vi "WVDIAL_1_MCSC_v1.vi"() -> ()   [LabVIEW 2012]
uses:
  <vilib>/Analysis/baseanly.llb/Mean (DBL).vi
  H2O_DIAL/LabVIEW-2012/Scalar_Data.vi
  AmcsUsb.dll
  <vilib>/Analysis/NI_AALBase.lvlib
panel:
  in  "Near Ch Offline mult":dbl=2.6
  in  "Data Reads":i32=770
  out "Loop Count":i32=770
  in  "TC Start":i32=100 min=1 max=1894
  in  "TC Length":i32=190 min=100 max=1894
  out "Total Counts":cluster{dbl, dbl, dbl, dbl}(graph)={168433.0, 167767.0, 1145442.0, 1147692.0}
  out "return type":i32
  out "Raw Uncorrected Return":dbl[][](graph)=[[20897.0, 17907.0, 61299.0, 1003.0, 932.0, 983.0, 951.0, 944.0, 1016.0, 1068.0, 1049.0, 1010.0, 1053.0, 979.0, 1043.0, 1051.0, 1088.0, 1105.0, 1050.0, 1051.0, 1029.0, 1012.0, 1012.0, 1067.0, 1114.0, 1055.0, 993.0, 1021.0, 944.0, 1017.0, 1050.0, 1058.0, 988.0, 1006.0, 985.0, 995.0, 1349.0, 2765.0, 4753.0, 5334.0, 4567.0, 3771.0, 2737.0, 1942.0, 1415.0, 1577.0, 1781.0, 1958.0, 1989.0, 1616.0, 5808.0, 11417.0, 8373.0, 1568.0, 979.0, 935.0, 900.0, 910.0, 923.0, 946.0, 962.0, 941.0, 927.0, 963.0, 943.0, 965.0, 941.0, 987.0, 993.0, 1007.0, 1151.0, 1083.0, 982.0, 1005.0, 997.0, 1039.0, 986.0, 980.0, 893.0, 968.0, 991.0, 1035.0, 1066.0, 1129.0, 1065.0, 1035.0, 926.0, 1000.0, 1000.0, 976.0, 914.0, 944.0, 888.0, 970.0, 917.0, 937.0, 943.0, 953.0, 866.0, 863.0, 952.0, 900.0, 961.0, 913.0, 941.0, 971.0, 946.0, 917.0, 939.0, 926.0, 944.0, 975.0, 937.0, 915.0, 916.0, 892.0, 900.0, 955.0, 938.0, 902.0, 912.0, 961.0, 927.0, 893.0, 938.0, 950.0, 882.0, 872.0, 953.0, 967.0, 902.0, 955.0, 932.0, 912.0, 969.0, 955.0, 951.0, 945.0, 994.0, 952.0, 949.0, 977.0, 917.0, 930.0, 888.0, 951.0, 935.0, 896.0, 923.0, 863.0, 979.0, 900.0, 1008.0, 893.0, 929.0, 917.0, 920.0, 943.0, 949.0, 881.0, 981.0, 916.0, 937.0, 911.0, 932.0, 945.0, 976.0, 882.0, 911.0, 994.0, 969.0, 919.0, 971.0, 898.0, 923.0, 930.0, 947.0, 904.0, 982.0, 933.0, 914.0, 970.0, 977.0, 881.0, 959.0, 947.0, 899.0, 949.0, 942.0, 951.0, 919.0, 910.0, 944.0, 931.0, 967.0, 901.0, 922.0, 921.0, 984.0, 977.0, 932.0, 906.0, 972.0, 872.0, 887.0, 920.0, 983.0, 1002.0, 945.0, 948.0, 897.0, 925.0, 965.0, 955.0, 909.0, 933.0, 953.0, 924.0, 972.0, 964.0, 961.0, 1002.0, 966.0, 904.0, 899.0, 951.0, 944.0, 938.0, 993.0, 893.0, 1016.0, 900.0, 879.0, 876.0, 944.0, 889.0, 935.0, 924.0, 961.0, 931.0, 933.0, 926.0, 862.0, 958.0, 885.0, 978.0, 968.0, 1002.0, 875.0, 912.0, 971.0, 922.0, 979.0, 959.0, 917.0, 971.0, 940.0, 891.0, 976.0, 932.0, 893.0, 934.0, 922.0, 989.0, 959.0, 932.0, 954.0, 947.0, 895.0, 950.0, 946.0, 943.0, 902.0, 911.0, 919.0, 1012.0, 904.0, 918.0, 965.0, 975.0], [922.0, 18275.0, 62214.0, 993.0, 957.0, 995.0, 1005.0, 1002.0, 1103.0, 1102.0, 1143.0, 1148.0, 1161.0, 1218.0, 1193.0, 1189.0, 1300.0, 1250.0, 1305.0, 1319.0, 1301.0, 1306.0, 1275.0, 1325.0, 1316.0, 1250.0, 1254.0, 1267.0, 1215.0, 1264.0, 1260.0, 1198.0, 1209.0, 1132.0, 1074.0, 1284.0, 2617.0, 7789.0, 14632.0, 16266.0, 14395.0, 11311.0, 8121.0, 5107.0, 3254.0, 3555.0, 4576.0, 5500.0, 5467.0, 4251.0, 20644.0, 36289.0, 27186.0, 3510.0, 957.0, 934.0, 965.0, 975.0, 950.0, 925.0, 944.0, 975.0, 978.0, 930.0, 906.0, 972.0, 923.0, 967.0, 1148.0, 1539.0, 1778.0, 1640.0, 1402.0, 1251.0, 1253.0, 1337.0, 1313.0, 1092.0, 1182.0, 1150.0, 1259.0, 1458.0, 1826.0, 1997.0, 1783.0, 1387.0, 1119.0, 1085.0, 1015.0, 951.0, 912.0, 947.0, 945.0, 935.0, 941.0, 910.0, 901.0, 897.0, 904.0, 895.0, 947.0, 962.0, 900.0, 1009.0, 902.0, 929.0, 908.0, 957.0, 926.0, 962.0, 886.0, 920.0, 978.0, 851.0, 975.0, 885.0, 895.0, 891.0, 932.0, 945.0, 937.0, 949.0, 907.0, 961.0, 933.0, 943.0, 921.0, 891.0, 970.0, 897.0, 927.0, 882.0, 911.0, 890.0, 918.0, 937.0, 944.0, 946.0, 946.0, 981.0, 967.0, 947.0, 969.0, 931.0, 967.0, 902.0, 946.0, 943.0, 987.0, 946.0, 945.0, 893.0, 956.0, 976.0, 955.0, 915.0, 885.0, 892.0, 921.0, 912.0, 952.0, 919.0, 940.0, 939.0, 959.0, 949.0, 943.0, 918.0, 927.0, 948.0, 965.0, 975.0, 926.0, 966.0, 963.0, 873.0, 939.0, 911.0, 911.0, 924.0, 904.0, 903.0, 944.0, 955.0, 928.0, 919.0, 934.0, 957.0, 907.0, 954.0, 901.0, 958.0, 897.0, 920.0, 899.0, 865.0, 891.0, 916.0, 938.0, 913.0, 918.0, 939.0, 921.0, 918.0, 917.0, 958.0, 931.0, 901.0, 962.0, 952.0, 909.0, 973.0, 910.0, 938.0, 927.0, 875.0, 909.0, 929.0, 944.0, 889.0, 910.0, 954.0, 882.0, 1028.0, 930.0, 964.0, 972.0, 955.0, 884.0, 897.0, 982.0, 990.0, 950.0, 997.0, 944.0, 923.0, 959.0, 932.0, 940.0, 881.0, 939.0, 911.0, 882.0, 939.0, 915.0, 910.0, 954.0, 900.0, 901.0, 917.0, 893.0, 923.0, 856.0, 962.0, 948.0, 949.0, 936.0, 912.0, 993.0, 946.0, 925.0, 947.0, 907.0, 942.0, 919.0, 960.0, 938.0, 910.0, 970.0, 926.0, 918.0, 977.0, 913.0, 956.0, 1017.0, 914.0, 896.0, 967.0, 958.0, 971.0], [901.0, 17238.0, 63738.0, 6571.0, 6627.0, 6967.0, 7037.0, 6952.0, 7011.0, 7085.0, 6916.0, 6955.0, 6689.0, 6750.0, 6599.0, 6621.0, 6454.0, 6505.0, 6415.0, 6424.0, 6268.0, 6518.0, 6408.0, 6477.0, 6500.0, 6370.0, 6334.0, 6434.0, 6392.0, 6309.0, 6236.0, 6430.0, 6473.0, 6304.0, 6382.0, 6382.0, 6442.0, 6892.0, 7617.0, 7974.0, 7667.0, 7436.0, 6895.0, 6739.0, 6455.0, 6647.0, 6742.0, 6717.0, 6663.0, 6624.0, 8201.0, 10372.0, 9200.0, 6714.0, 6266.0, 6292.0, 6417.0, 6314.0, 6468.0, 6234.0, 6317.0, 6307.0, 6331.0, 6281.0, 6488.0, 6596.0, 6326.0, 6351.0, 6400.0, 6372.0, 6588.0, 6340.0, 6501.0, 6412.0, 6397.0, 6327.0, 6430.0, 6407.0, 6300.0, 6410.0, 6250.0, 6385.0, 6411.0, 6512.0, 6402.0, 6362.0, 6367.0, 6405.0, 6382.0, 6281.0, 6268.0, 6347.0, 6348.0, 6282.0, 6292.0, 6409.0, 6275.0, 6302.0, 6415.0, 6451.0, 6367.0, 6295.0, 6437.0, 6473.0, 6337.0, 6355.0, 6512.0, 6531.0, 6283.0, 6269.0, 6368.0, 6344.0, 6443.0, 6369.0, 6353.0, 6385.0, 6425.0, 6409.0, 6377.0, 6322.0, 6353.0, 6410.0, 6508.0, 6432.0, 6298.0, 6322.0, 6420.0, 6301.0, 6325.0, 6279.0, 6361.0, 6224.0, 6237.0, 6273.0, 6424.0, 6416.0, 6355.0, 6469.0, 6373.0, 6349.0, 6311.0, 6368.0, 6282.0, 6355.0, 6237.0, 6397.0, 6338.0, 6287.0, 6364.0, 6378.0, 6295.0, 6332.0, 6342.0, 6137.0, 6260.0, 6253.0, 6331.0, 6303.0, 6393.0, 6325.0, 6329.0, 6517.0, 6423.0, 6344.0, 6284.0, 6385.0, 6362.0, 6389.0, 6357.0, 6402.0, 6446.0, 6402.0, 6361.0, 6328.0, 6470.0, 6458.0, 6454.0, 6466.0, 6453.0, 6293.0, 6483.0, 6398.0, 6271.0, 6379.0, 6351.0, 6323.0, 6291.0, 6350.0, 6366.0, 6509.0, 6445.0, 6334.0, 6295.0, 6337.0, 6310.0, 6311.0, 6417.0, 6356.0, 6309.0, 6411.0, 6380.0, 6260.0, 6532.0, 6352.0, 6394.0, 6461.0, 6402.0, 6391.0, 6400.0, 6353.0, 6339.0, 6360.0, 6365.0, 6437.0, 6335.0, 6297.0, 6511.0, 6365.0, 6283.0, 6384.0, 6464.0, 6297.0, 6291.0, 6346.0, 6384.0, 6355.0, 6530.0, 6417.0, 6334.0, 6364.0, 6340.0, 6344.0, 6367.0, 6388.0, 6356.0, 6285.0, 6258.0, 6281.0, 6322.0, 6328.0, 6406.0, 6450.0, 6343.0, 6354.0, 6275.0, 6425.0, 6245.0, 6236.0, 6392.0, 6339.0, 6318.0, 6406.0, 6458.0, 6358.0, 6344.0, 6388.0, 6304.0, 6356.0, 6277.0, 6408.0, 6439.0, 6308.0, 6440.0, 6412.0, 6283.0, 6365.0, 6320.0, 6403.0, 6318.0, 6412.0, 6326.0, 6403.0, 6439.0, 6369.0, 6437.0, 6351.0, 6319.0, 6382.0, 6454.0, 6288.0], [6387.0, 17467.0, 65418.0, 6569.0, 6883.0, 7052.0, 7265.0, 7267.0, 7422.0, 7428.0, 7449.0, 7216.0, 7212.0, 7028.0, 7067.0, 6796.0, 6717.0, 6721.0, 6668.0, 6585.0, 6511.0, 6639.0, 6441.0, 6629.0, 6525.0, 6450.0, 6456.0, 6381.0, 6453.0, 6451.0, 6380.0, 6479.0, 6424.0, 6473.0, 6587.0, 6463.0, 6806.0, 8963.0, 11686.0, 12297.0, 11494.0, 10217.0, 8973.0, 7870.0, 7087.0, 7226.0, 7776.0, 8067.0, 7957.0, 7562.0, 14612.0, 22974.0, 18051.0, 7202.0, 6396.0, 6350.0, 6276.0, 6334.0, 6252.0, 6328.0, 6420.0, 6377.0, 6390.0, 6417.0, 6109.0, 6349.0, 6440.0, 6362.0, 6392.0, 6574.0, 6721.0, 6603.0, 6431.0, 6561.0, 6489.0, 6579.0, 6553.0, 6384.0, 6426.0, 6566.0, 6460.0, 6546.0, 6644.0, 6799.0, 6611.0, 6466.0, 6404.0, 6440.0, 6429.0, 6422.0, 6470.0, 6469.0, 6344.0, 6403.0, 6356.0, 6332.0, 6325.0, 6357.0, 6387.0, 6302.0, 6368.0, 6319.0, 6370.0, 6280.0, 6314.0, 6284.0, 6539.0, 6299.0, 6473.0, 6404.0, 6434.0, 6321.0, 6398.0, 6364.0, 6362.0, 6331.0, 6194.0, 6478.0, 6333.0, 6361.0, 6353.0, 6462.0, 6312.0, 6339.0, 6442.0, 6356.0, 6323.0, 6326.0, 6156.0, 6417.0, 6400.0, 6307.0, 6432.0, 6475.0, 6443.0, 6344.0, 6491.0, 6349.0, 6424.0, 6413.0, 6400.0, 6355.0, 6257.0, 6390.0, 6370.0, 6310.0, 6401.0, 6381.0, 6368.0, 6334.0, 6345.0, 6308.0, 6398.0, 6468.0, 6360.0, 6383.0, 6282.0, 6362.0, 6426.0, 6223.0, 6353.0, 6331.0, 6316.0, 6430.0, 6376.0, 6238.0, 6391.0, 6473.0, 6431.0, 6212.0, 6449.0, 6320.0, 6221.0, 6424.0, 6517.0, 6326.0, 6446.0, 6387.0, 6435.0, 6374.0, 6360.0, 6343.0, 6251.0, 6365.0, 6487.0, 6334.0, 6413.0, 6253.0, 6326.0, 6380.0, 6443.0, 6296.0, 6362.0, 6364.0, 6433.0, 6391.0, 6366.0, 6352.0, 6388.0, 6283.0, 6323.0, 6363.0, 6510.0, 6479.0, 6381.0, 6344.0, 6254.0, 6469.0, 6362.0, 6480.0, 6281.0, 6354.0, 6394.0, 6356.0, 6462.0, 6302.0, 6447.0, 6399.0, 6375.0, 6278.0, 6288.0, 6376.0, 6356.0, 6356.0, 6525.0, 6377.0, 6346.0, 6397.0, 6259.0, 6405.0, 6298.0, 6418.0, 6367.0, 6332.0, 6368.0, 6431.0, 6486.0, 6306.0, 6475.0, 6464.0, 6203.0, 6377.0, 6447.0, 6446.0, 6348.0, 6434.0, 6307.0, 6351.0, 6433.0, 6453.0, 6390.0, 6584.0, 6449.0, 6479.0, 6440.0, 6412.0, 6408.0, 6425.0, 6520.0, 6380.0, 6473.0, 6278.0, 6354.0, 6331.0, 6376.0, 6455.0, 6498.0, 6372.0, 6217.0, 6468.0, 6336.0, 6316.0, 6267.0, 6498.0, 6364.0, 6503.0, 6347.0, 6397.0, 6366.0, 6396.0]]
  in  "stop":bool
  out "Corrected Return":dbl[][](graph)=[[19959.617021276597, 16969.617021276597, 60361.617021276594, 65.61702127659578, -5.3829787234042215, 45.61702127659578, 13.617021276595779, 6.6170212765957785, 78.61702127659578, 130.61702127659578, 111.61702127659578, 72.61702127659578, 115.61702127659578, 41.61702127659578, 105.61702127659578, 113.61702127659578, 150.61702127659578, 167.61702127659578, 112.61702127659578, 113.61702127659578, 91.61702127659578, 74.61702127659578, 74.61702127659578, 129.61702127659578, 176.61702127659578, 117.61702127659578, 55.61702127659578, 83.61702127659578, 6.6170212765957785, 79.61702127659578, 112.61702127659578, 120.61702127659578, 50.61702127659578, 68.61702127659578, 47.61702127659578, 57.61702127659578, 411.6170212765958, 1827.6170212765958, 3815.6170212765956, 4396.617021276596, 3629.6170212765956, 2833.6170212765956, 1799.6170212765958, 1004.6170212765958, 477.6170212765958, 639.6170212765958, 843.6170212765958, 1020.6170212765958, 1051.6170212765958, 678.6170212765958, 4870.617021276596, 10479.617021276596, 7435.617021276596, 630.6170212765958, 41.61702127659578, -2.3829787234042215, -37.38297872340422, -27.38297872340422, -14.382978723404221, 8.617021276595779, 24.61702127659578, 3.6170212765957785, -10.382978723404221, 25.61702127659578, 5.6170212765957785, 27.61702127659578, 3.6170212765957785, 49.61702127659578, 55.61702127659578, 69.61702127659578, 213.61702127659578, 145.61702127659578, 44.61702127659578, 67.61702127659578, 59.61702127659578, 101.61702127659578, 48.61702127659578, 42.61702127659578, -44.38297872340422, 30.61702127659578, 53.61702127659578, 97.61702127659578, 128.61702127659578, 191.61702127659578, 127.61702127659578, 97.61702127659578, -11.382978723404221, 62.61702127659578, 62.61702127659578, 38.61702127659578, -23.38297872340422, 6.6170212765957785, -49.38297872340422, 32.61702127659578, -20.38297872340422, -0.38297872340422145, 5.6170212765957785, 15.617021276595779, -71.38297872340422, -74.38297872340422, 14.617021276595779, -37.38297872340422, 23.61702127659578, -24.38297872340422, 3.6170212765957785, 33.61702127659578, 8.617021276595779, -20.38297872340422, 1.6170212765957785, -11.382978723404221, 6.6170212765957785, 37.61702127659578, -0.38297872340422145, -22.38297872340422, -21.38297872340422, -45.38297872340422, -37.38297872340422, 17.61702127659578, 0.6170212765957785, -35.38297872340422, -25.38297872340422, 23.61702127659578, -10.382978723404221, -44.38297872340422, 0.6170212765957785, 12.617021276595779, -55.38297872340422, -65.38297872340422, 15.617021276595779, 29.61702127659578, -35.38297872340422, 17.61702127659578, -5.3829787234042215, -25.38297872340422, 31.61702127659578, 17.61702127659578, 13.617021276595779, 7.6170212765957785, 56.61702127659578, 14.617021276595779, 11.617021276595779, 39.61702127659578, -20.38297872340422, -7.3829787234042215, -49.38297872340422, 13.617021276595779, -2.3829787234042215, -41.38297872340422, -14.382978723404221, -74.38297872340422, 41.61702127659578, -37.38297872340422, 70.61702127659578, -44.38297872340422, -8.382978723404221, -20.38297872340422, -17.38297872340422, 5.6170212765957785, 11.617021276595779, -56.38297872340422, 43.61702127659578, -21.38297872340422, -0.38297872340422145, -26.38297872340422, -5.3829787234042215, 7.6170212765957785, 38.61702127659578, -55.38297872340422, -26.38297872340422, 56.61702127659578, 31.61702127659578, -18.38297872340422, 33.61702127659578, -39.38297872340422, -14.382978723404221, -7.3829787234042215, 9.617021276595779, -33.38297872340422, 44.61702127659578, -4.3829787234042215, -23.38297872340422, 32.61702127659578, 39.61702127659578, -56.38297872340422, 21.61702127659578, 9.617021276595779, -38.38297872340422, 11.617021276595779, 4.6170212765957785, 13.617021276595779, -18.38297872340422, -27.38297872340422, 6.6170212765957785, -6.3829787234042215, 29.61702127659578, -36.38297872340422, -15.382978723404221, -16.38297872340422, 46.61702127659578, 39.61702127659578, -5.3829787234042215, -31.38297872340422, 34.61702127659578, -65.38297872340422, -50.38297872340422, -17.38297872340422, 45.61702127659578, 64.61702127659578, 7.6170212765957785, 10.617021276595779, -40.38297872340422, -12.382978723404221, 27.61702127659578, 17.61702127659578, -28.38297872340422, -4.3829787234042215, 15.617021276595779, -13.382978723404221, 34.61702127659578, 26.61702127659578, 23.61702127659578, 64.61702127659578, 28.61702127659578, -33.38297872340422, -38.38297872340422, 13.617021276595779, 6.6170212765957785, 0.6170212765957785, 55.61702127659578, -44.38297872340422, 78.61702127659578, -37.38297872340422, -58.38297872340422, -61.38297872340422, 6.6170212765957785, -48.38297872340422, -2.3829787234042215, -13.382978723404221, 23.61702127659578, -6.3829787234042215, -4.3829787234042215, -11.382978723404221, -75.38297872340422, 20.61702127659578, -52.38297872340422, 40.61702127659578, 30.61702127659578, 64.61702127659578, -62.38297872340422, -25.38297872340422, 33.61702127659578, -15.382978723404221, 41.61702127659578, 21.61702127659578, -20.38297872340422, 33.61702127659578, 2.6170212765957785, -46.38297872340422, 38.61702127659578, -5.3829787234042215, -44.38297872340422, -3.3829787234042215, -15.382978723404221, 51.61702127659578, 21.61702127659578, -5.3829787234042215, 16.61702127659578, 9.617021276595779, -42.38297872340422, 12.617021276595779, 8.617021276595779, 5.6170212765957785, -35.38297872340422, -26.38297872340422, -18.38297872340422, 74.61702127659578, -33.38297872340422, -19.38297872340422, 27.61702127659578, 37.61702127659578], [-9.5, 17343.5, 61282.5, 61.5, 25.5, 63.5, 73.5, 70.5, 171.5, 170.5, 211.5, 216.5, 229.5, 286.5, 261.5, 257.5, 368.5, 318.5, 373.5, 387.5, 369.5, 374.5, 343.5, 393.5, 384.5, 318.5, 322.5, 335.5, 283.5, 332.5, 328.5, 266.5, 277.5, 200.5, 142.5, 352.5, 1685.5, 6857.5, 13700.5, 15334.5, 13463.5, 10379.5, 7189.5, 4175.5, 2322.5, 2623.5, 3644.5, 4568.5, 4535.5, 3319.5, 19712.5, 35357.5, 26254.5, 2578.5, 25.5, 2.5, 33.5, 43.5, 18.5, -6.5, 12.5, 43.5, 46.5, -1.5, -25.5, 40.5, -8.5, 35.5, 216.5, 607.5, 846.5, 708.5, 470.5, 319.5, 321.5, 405.5, 381.5, 160.5, 250.5, 218.5, 327.5, 526.5, 894.5, 1065.5, 851.5, 455.5, 187.5, 153.5, 83.5, 19.5, -19.5, 15.5, 13.5, 3.5, 9.5, -21.5, -30.5, -34.5, -27.5, -36.5, 15.5, 30.5, -31.5, 77.5, -29.5, -2.5, -23.5, 25.5, -5.5, 30.5, -45.5, -11.5, 46.5, -80.5, 43.5, -46.5, -36.5, -40.5, 0.5, 13.5, 5.5, 17.5, -24.5, 29.5, 1.5, 11.5, -10.5, -40.5, 38.5, -34.5, -4.5, -49.5, -20.5, -41.5, -13.5, 5.5, 12.5, 14.5, 14.5, 49.5, 35.5, 15.5, 37.5, -0.5, 35.5, -29.5, 14.5, 11.5, 55.5, 14.5, 13.5, -38.5, 24.5, 44.5, 23.5, -16.5, -46.5, -39.5, -10.5, -19.5, 20.5, -12.5, 8.5, 7.5, 27.5, 17.5, 11.5, -13.5, -4.5, 16.5, 33.5, 43.5, -5.5, 34.5, 31.5, -58.5, 7.5, -20.5, -20.5, -7.5, -27.5, -28.5, 12.5, 23.5, -3.5, -12.5, 2.5, 25.5, -24.5, 22.5, -30.5, 26.5, -34.5, -11.5, -32.5, -66.5, -40.5, -15.5, 6.5, -18.5, -13.5, 7.5, -10.5, -13.5, -14.5, 26.5, -0.5, -30.5, 30.5, 20.5, -22.5, 41.5, -21.5, 6.5, -4.5, -56.5, -22.5, -2.5, 12.5, -42.5, -21.5, 22.5, -49.5, 96.5, -1.5, 32.5, 40.5, 23.5, -47.5, -34.5, 50.5, 58.5, 18.5, 65.5, 12.5, -8.5, 27.5, 0.5, 8.5, -50.5, 7.5, -20.5, -49.5, 7.5, -16.5, -21.5, 22.5, -31.5, -30.5, -14.5, -38.5, -8.5, -75.5, 30.5, 16.5, 17.5, 4.5, -19.5, 61.5, 14.5, -6.5, 15.5, -24.5, 10.5, -12.5, 28.5, 6.5, -21.5, 38.5, -5.5, -13.5, 45.5, -18.5, 24.5, 85.5, -17.5, -35.5, 35.5, 26.5, 39.5], [-14204.546808510639, 28271.653191489364, 149171.65319148937, 537.4531914893626, 683.0531914893626, 1567.0531914893625, 1749.0531914893625, 1528.0531914893625, 1681.4531914893626, 1873.8531914893626, 1434.4531914893626, 1535.8531914893626, 844.2531914893625, 1002.8531914893625, 610.2531914893625, 667.4531914893626, 233.2531914893625, 365.85319148936253, 131.8531914893625, 155.2531914893625, -250.34680851063752, 399.65319148936254, 113.65319148936251, 293.0531914893625, 352.85319148936253, 14.853191489362507, -78.74680851063749, 181.2531914893625, 72.0531914893625, -143.7468085106375, -333.5468085106375, 170.8531914893625, 282.65319148936254, -156.7468085106375, 46.05319148936251, 46.05319148936251, 202.05319148936252, 1372.0531914893625, 3257.0531914893627, 4185.2531914893625, 3387.0531914893627, 2786.453191489363, 1379.8531914893626, 974.2531914893625, 235.8531914893625, 735.0531914893626, 982.0531914893626, 917.0531914893626, 776.6531914893625, 675.2531914893625, 4775.453191489362, 10420.053191489364, 7372.853191489363, 909.2531914893625, -255.5468085106375, -187.9468085106375, 137.05319148936252, -130.7468085106375, 269.65319148936254, -338.7468085106375, -122.9468085106375, -148.9468085106375, -86.54680851063749, -216.5468085106375, 321.65319148936254, 602.4531914893626, -99.54680851063749, -34.5468085106375, 92.85319148936252, 20.053191489362508, 581.6531914893625, -63.1468085106375, 355.4531914893625, 124.0531914893625, 85.0531914893625, -96.9468085106375, 170.8531914893625, 111.0531914893625, -167.1468085106375, 118.85319148936252, -297.1468085106375, 53.85319148936251, 121.45319148936251, 384.0531914893625, 98.0531914893625, -5.946808510637493, 7.053191489362507, 105.85319148936252, 46.05319148936251, -216.5468085106375, -250.34680851063752, -44.946808510637496, -42.346808510637494, -213.9468085106375, -187.9468085106375, 116.25319148936251, -232.1468085106375, -161.9468085106375, 131.8531914893625, 225.45319148936252, 7.053191489362507, -180.1468085106375, 189.05319148936252, 282.65319148936254, -70.9468085106375, -24.146808510637495, 384.0531914893625, 433.4531914893625, -211.3468085106375, -247.7468085106375, 9.653191489362507, -52.74680851063749, 204.6531914893625, 12.253191489362507, -29.346808510637494, 53.85319148936251, 157.8531914893625, 116.25319148936251, 33.05319148936251, -109.9468085106375, -29.346808510637494, 118.85319148936252, 373.65319148936254, 176.05319148936252, -172.3468085106375, -109.9468085106375, 144.8531914893625, -164.5468085106375, -102.1468085106375, -221.7468085106375, -8.546808510637494, -364.7468085106375, -330.9468085106375, -237.3468085106375, 155.2531914893625, 134.45319148936252, -24.146808510637495, 272.2531914893625, 22.65319148936251, -39.74680851063749, -138.5468085106375, 9.653191489362507, -213.9468085106375, -24.146808510637495, -330.9468085106375, 85.0531914893625, -68.3468085106375, -200.9468085106375, -0.7468085106374929, 35.653191489362506, -180.1468085106375, -83.9468085106375, -57.946808510637496, -590.9468085106375, -271.1468085106375, -289.3468085106375, -86.54680851063749, -159.3468085106375, 74.65319148936251, -102.1468085106375, -91.74680851063749, 397.0531914893625, 152.6531914893625, -52.74680851063749, -208.7468085106375, 53.85319148936251, -5.946808510637493, 64.25319148936251, -18.946808510637492, 98.0531914893625, 212.45319148936252, 98.0531914893625, -8.546808510637494, -94.3468085106375, 274.85319148936253, 243.6531914893625, 233.2531914893625, 264.4531914893625, 230.6531914893625, -185.3468085106375, 308.65319148936254, 87.65319148936251, -242.5468085106375, 38.25319148936251, -34.5468085106375, -107.3468085106375, -190.5468085106375, -37.14680851063749, 4.453191489362507, 376.2531914893625, 209.8531914893625, -78.74680851063749, -180.1468085106375, -70.9468085106375, -141.1468085106375, -138.5468085106375, 137.05319148936252, -21.546808510637494, -143.7468085106375, 121.45319148936251, 40.85319148936251, -271.1468085106375, 436.0531914893625, -31.946808510637496, 77.25319148936251, 251.45319148936252, 98.0531914893625, 69.45319148936251, 92.85319148936252, -29.346808510637494, -65.74680851063749, -11.146808510637493, 1.8531914893625072, 189.05319148936252, -76.1468085106375, -174.9468085106375, 381.4531914893625, 1.8531914893625072, -211.3468085106375, 51.25319148936251, 259.2531914893625, -174.9468085106375, -190.5468085106375, -47.5468085106375, 51.25319148936251, -24.146808510637495, 430.85319148936253, 137.05319148936252, -78.74680851063749, -0.7468085106374929, -63.1468085106375, -52.74680851063749, 7.053191489362507, 61.653191489362506, -21.546808510637494, -206.1468085106375, -276.3468085106375, -216.5468085106375, -109.9468085106375, -94.3468085106375, 108.45319148936251, 222.8531914893625, -55.346808510637494, -26.746808510637493, -232.1468085106375, 157.8531914893625, -310.1468085106375, -333.5468085106375, 72.0531914893625, -65.74680851063749, -120.3468085106375, 108.45319148936251, 243.6531914893625, -16.346808510637494, -52.74680851063749, 61.653191489362506, -156.7468085106375, -21.546808510637494, -226.9468085106375, 113.65319148936251, 194.2531914893625, -146.3468085106375, 196.8531914893625, 124.0531914893625, -211.3468085106375, 1.8531914893625072, -115.1468085106375, 100.65319148936251, -120.3468085106375, 124.0531914893625, -99.54680851063749, 100.65319148936251, 194.2531914893625, 12.253191489362507, 189.05319148936252, -34.5468085106375, -117.74680851063749, 46.05319148936251, 233.2531914893625, -198.3468085106375], [5.172340425532821, 28813.172340425535, 153485.77234042555, 478.37234042553285, 1294.7723404255328, 1734.1723404255329, 2287.972340425533, 2293.172340425533, 2696.172340425533, 2711.772340425533, 2766.372340425533, 2160.5723404255327, 2150.172340425533, 1671.7723404255328, 1773.1723404255329, 1068.572340425533, 863.1723404255329, 873.5723404255328, 735.7723404255329, 519.9723404255328, 327.57234042553284, 660.3723404255328, 145.57234042553281, 634.3723404255328, 363.9723404255328, 168.97234042553282, 184.57234042553281, -10.42765957446718, 176.77234042553283, 171.57234042553281, -13.02765957446718, 244.37234042553283, 101.37234042553283, 228.77234042553283, 525.1723404255329, 202.77234042553283, 1094.572340425533, 6702.772340425533, 13782.572340425533, 15371.172340425534, 13283.372340425532, 9963.172340425534, 6728.772340425533, 3860.972340425533, 1825.1723404255329, 2186.5723404255327, 3616.5723404255327, 4373.172340425533, 4087.172340425533, 3060.172340425533, 21390.172340425535, 43131.372340425536, 30331.572340425533, 2124.172340425533, 28.572340425532822, -91.02765957446718, -283.4276595744672, -132.62765957446717, -345.8276595744672, -148.2276595744672, 90.97234042553282, -20.82765957446718, 12.97234042553282, 83.17234042553282, -717.6276595744672, -93.62765957446719, 142.97234042553282, -59.827659574467184, 18.17234042553282, 491.37234042553285, 873.5723404255328, 566.7723404255329, 119.57234042553283, 457.57234042553284, 270.37234042553285, 504.37234042553285, 436.77234042553283, -2.6276595744671796, 106.57234042553283, 470.57234042553284, 194.97234042553282, 418.57234042553284, 673.3723404255328, 1076.372340425533, 587.5723404255328, 210.57234042553281, 49.37234042553282, 142.97234042553282, 114.37234042553283, 96.17234042553282, 220.97234042553282, 218.37234042553283, -106.62765957446719, 46.772340425532825, -75.42765957446719, -137.8276595744672, -156.02765957446718, -72.82765957446718, 5.172340425532821, -215.8276595744672, -44.22765957446718, -171.62765957446717, -39.02765957446718, -273.0276595744672, -184.62765957446717, -262.6276595744672, 400.37234042553285, -223.62765957446717, 228.77234042553283, 49.37234042553282, 127.37234042553283, -166.42765957446719, 33.772340425532825, -54.62765957446718, -59.827659574467184, -140.42765957446719, -496.6276595744672, 241.77234042553283, -135.2276595744672, -62.427659574467185, -83.22765957446718, 200.17234042553284, -189.8276595744672, -119.62765957446719, 148.17234042553284, -75.42765957446719, -161.2276595744672, -153.42765957446719, -595.4276595744672, 83.17234042553282, 38.97234042553282, -202.8276595744672, 122.17234042553282, 233.97234042553282, 150.77234042553283, -106.62765957446719, 275.57234042553284, -93.62765957446719, 101.37234042553283, 72.77234042553282, 38.97234042553282, -78.02765957446718, -332.8276595744672, 12.97234042553282, -39.02765957446718, -195.02765957446718, 41.57234042553282, -10.42765957446718, -44.22765957446718, -132.62765957446717, -104.02765957446718, -200.2276595744672, 33.772340425532825, 215.77234042553283, -65.02765957446718, -5.22765957446718, -267.8276595744672, -59.827659574467184, 106.57234042553283, -421.22765957446717, -83.22765957446718, -140.42765957446719, -179.42765957446719, 116.97234042553282, -23.42765957446718, -382.22765957446717, 15.57234042553282, 228.77234042553283, 119.57234042553283, -449.8276595744672, 166.37234042553283, -169.02765957446718, -426.4276595744672, 101.37234042553283, 343.1723404255328, -153.42765957446719, 158.57234042553281, 5.172340425532821, 129.97234042553282, -28.62765957446718, -65.02765957446718, -109.22765957446718, -348.4276595744672, -52.02765957446718, 265.1723404255328, -132.62765957446717, 72.77234042553282, -343.22765957446717, -153.42765957446719, -13.02765957446718, 150.77234042553283, -231.42765957446719, -59.827659574467184, -54.62765957446718, 124.77234042553282, 15.57234042553282, -49.42765957446718, -85.82765957446718, 7.77234042553282, -265.22765957446717, -161.2276595744672, -57.22765957446718, 324.9723404255328, 244.37234042553283, -10.42765957446718, -106.62765957446719, -340.6276595744672, 218.37234042553283, -59.827659574467184, 246.97234042553282, -270.4276595744672, -80.62765957446719, 23.372340425532823, -75.42765957446719, 200.17234042553284, -215.8276595744672, 161.17234042553284, 36.37234042553282, -26.02765957446718, -278.22765957446717, -252.2276595744672, -23.42765957446718, -75.42765957446719, -75.42765957446719, 363.9723404255328, -20.82765957446718, -101.42765957446719, 31.17234042553282, -327.6276595744672, 51.97234042553282, -226.2276595744672, 85.77234042553282, -46.827659574467184, -137.8276595744672, -44.22765957446718, 119.57234042553283, 262.57234042553284, -205.42765957446719, 233.97234042553282, 205.37234042553283, -473.22765957446717, -20.82765957446718, 161.17234042553284, 158.57234042553281, -96.22765957446718, 127.37234042553283, -202.8276595744672, -88.42765957446719, 124.77234042553282, 176.77234042553283, 12.97234042553282, 517.3723404255328, 166.37234042553283, 244.37234042553283, 142.97234042553282, 70.17234042553282, 59.772340425532825, 103.97234042553282, 350.9723404255328, -13.02765957446718, 228.77234042553283, -278.22765957446717, -80.62765957446719, -140.42765957446719, -23.42765957446718, 181.97234042553282, 293.77234042553283, -33.827659574467184, -436.8276595744672, 215.77234042553283, -127.42765957446719, -179.42765957446719, -306.8276595744672, 293.77234042553283, -54.62765957446718, 306.77234042553283, -98.82765957446718, 31.17234042553282, -49.42765957446718, 28.572340425532822]] caption="Corrected Signal"
  out "Max. Rep. Rate (Hz)":dbl=7091.695624423801
  out "Data Collection Time per Column":dbl=1.4001
  out "Minimum Sync Pulse Period(µs)":dbl=141.01 format="%.2f"
  in  "y units":u16(ring) items=["Bin #", "Sampling Time(µs)", "Range(m)"]
  in  "Time Resolution Per Bin(ns)":u16=500 min=5 max=1063 step=1
  in  "Number of Accumulates":u32=10000 min=1 max=32767 step=1
  in  "Number of Bins":u32=280 min=2 max=4095 step=1
  in  "Pulse A Polarity":enum16{"Low", "High"}(ring)=enum."High"
  in  "Sync Pulse Polarity":enum32{"Low", "High"}(ring)=enum."High"
  in  "Accumulation Delay(ns)":u16=10 min=10 max=1270 step=1
  in  "Pulse B Delay(ns)":u32=170000 min=80 max=327600 step=1
  in  "Pulse A Delay(ns)":u32=1040 min=80 max=327600
  in  "bins":u32=280 min=2 max=4095 step=1
  out "y offset":u16=10
  in  "ns scale":u16=500
  in  "Pulse B Polarity":enum16{"Low", "High"}(ring)=enum."High"
  out "Running?":bool
  out "Device ID":u32
  out "Open?":bool=TRUE
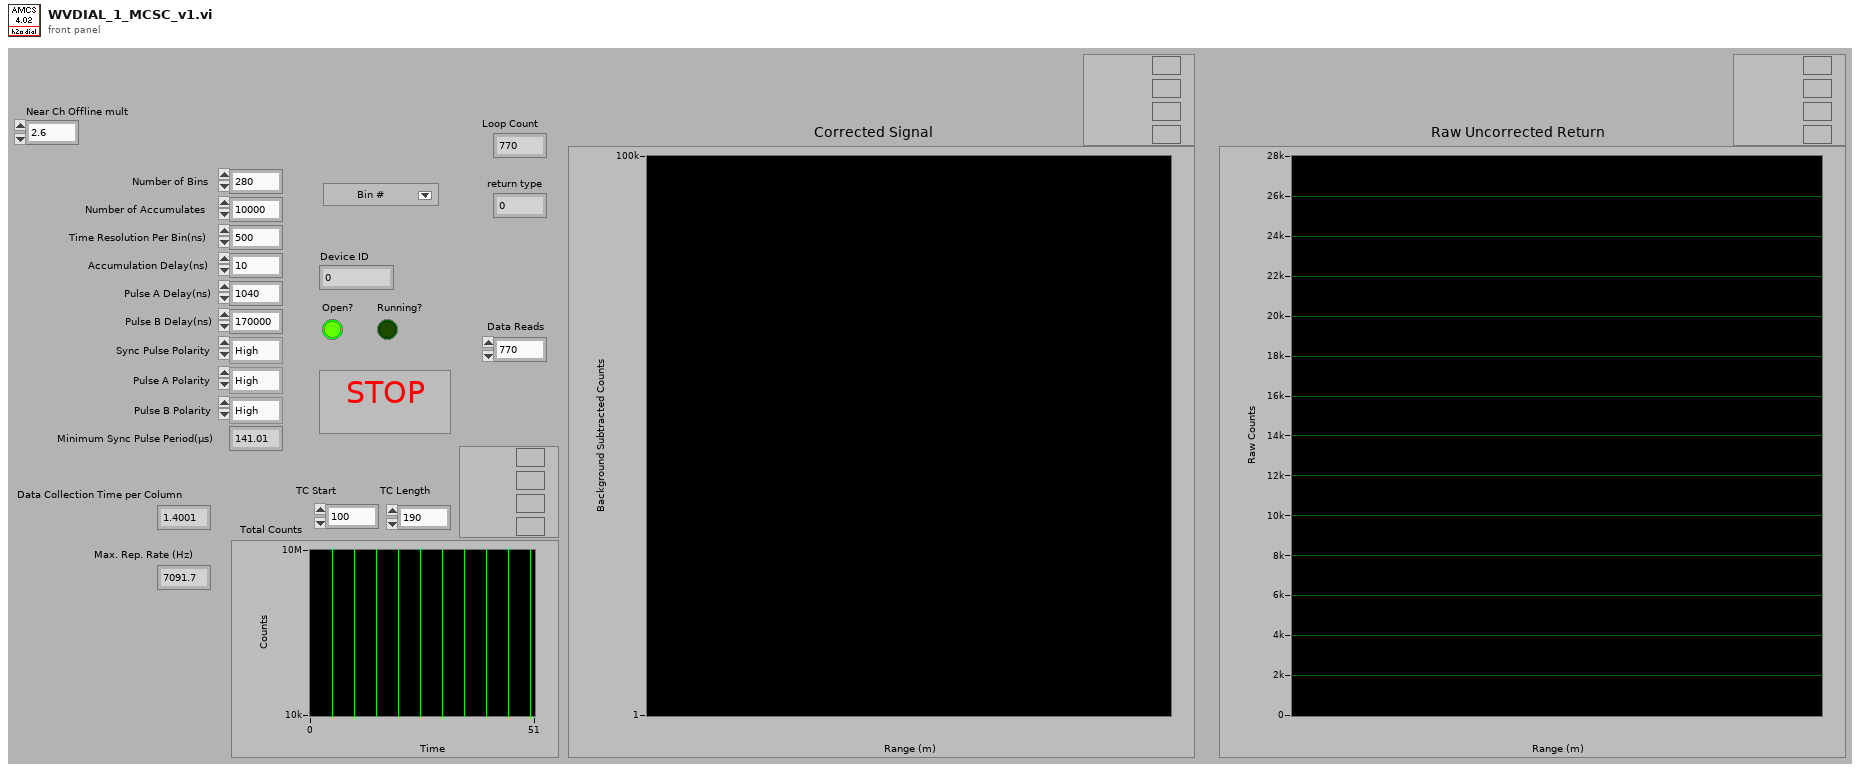
[diagram p1: front panel]
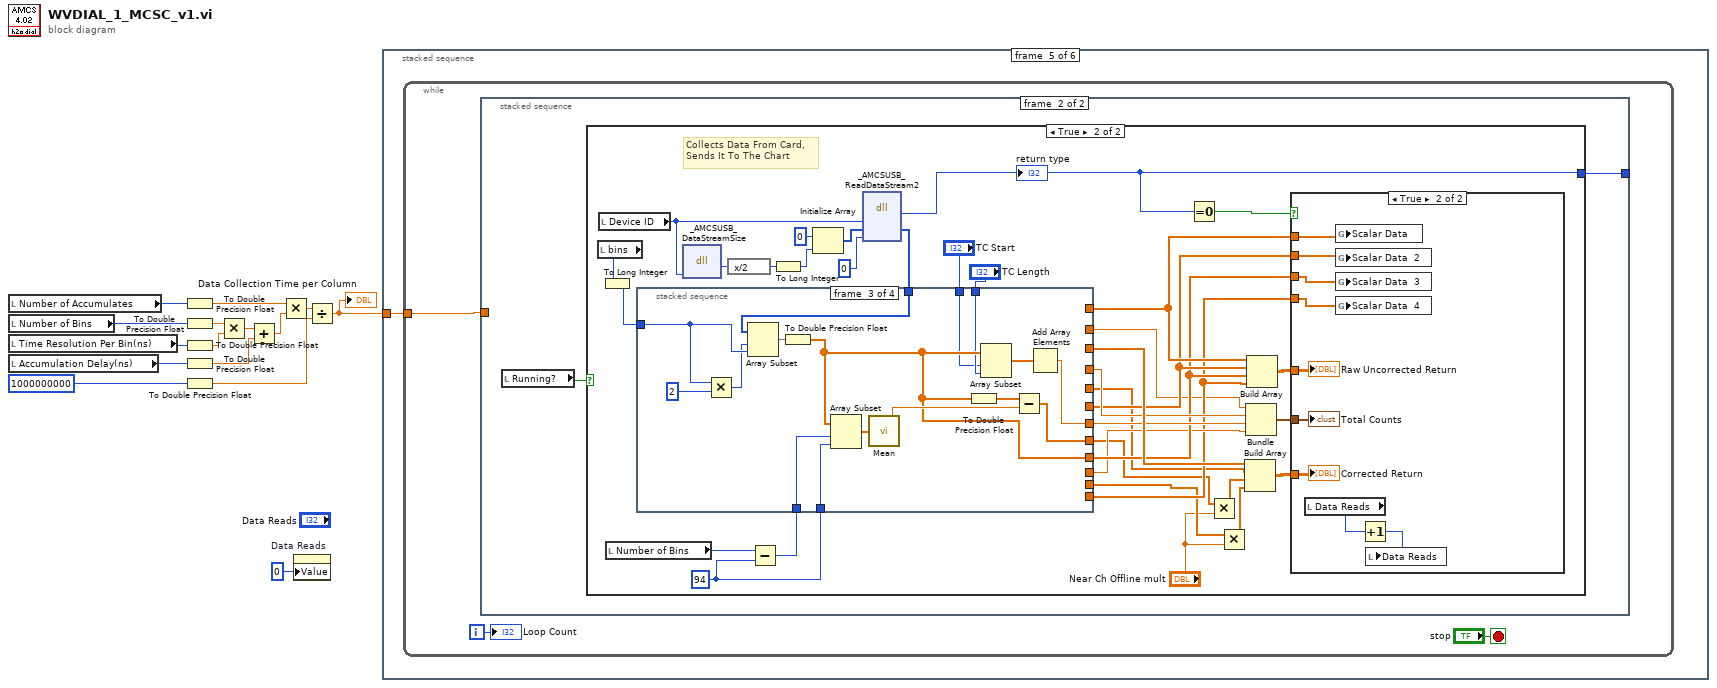
[diagram p0: block diagram]
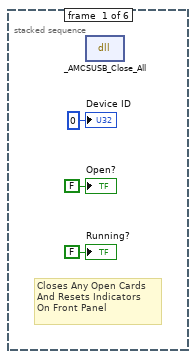
[diagram p2: hidden frame]
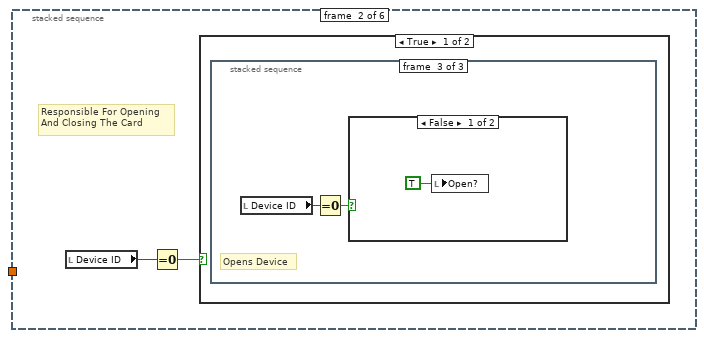
[diagram p3: hidden frame]
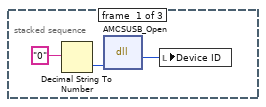
[diagram p4: hidden frame]
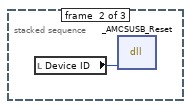
[diagram p5: hidden frame]
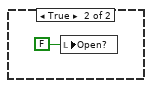
[diagram p6: hidden frame]
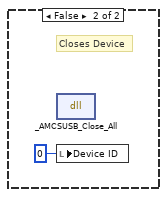
[diagram p7: hidden frame]
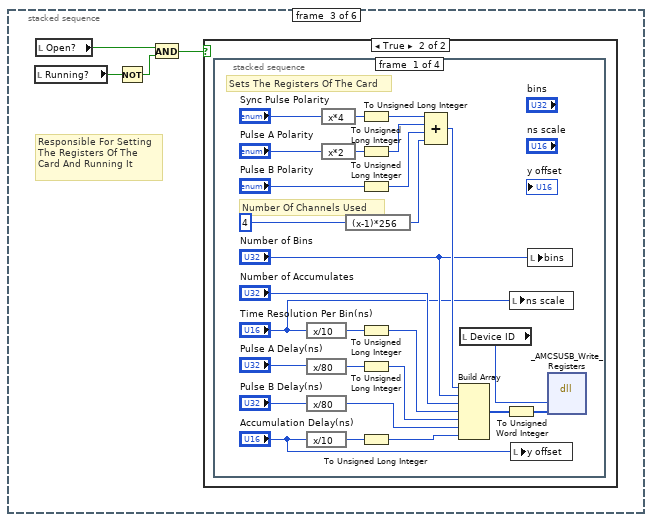
[diagram p8: hidden frame]
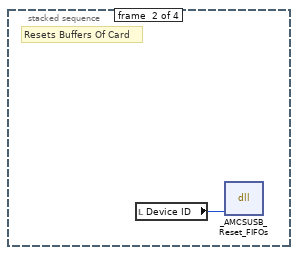
[diagram p10: hidden frame]
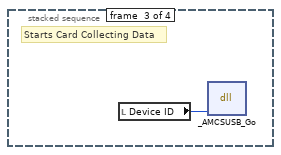
[diagram p11: hidden frame]
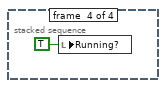
[diagram p12: hidden frame]
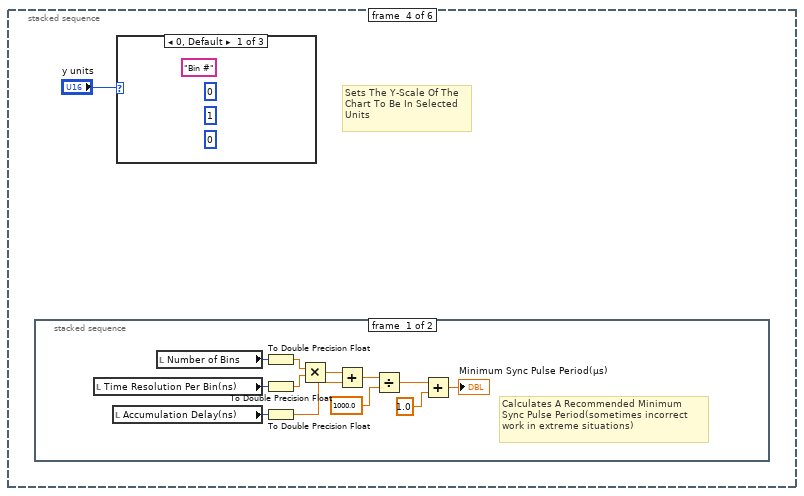
[diagram p13: hidden frame]
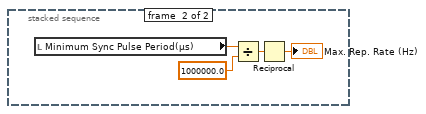
[diagram p14: hidden frame]
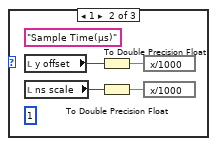
[diagram p15: hidden frame]
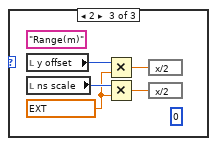
[diagram p16: hidden frame]
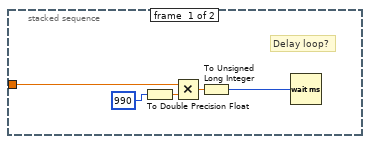
[diagram p17: hidden frame]
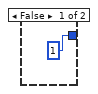
[diagram p18: hidden frame]
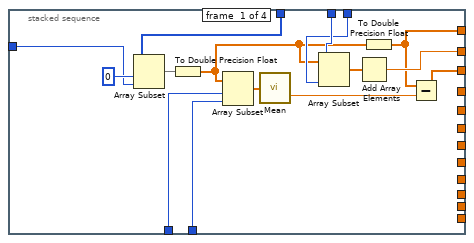
[diagram p20: hidden frame]
diagram:
  n1 = local read "Number of Accumulates"() -> (w11:u32)
  n2 = local read "Number of Bins"() -> (w6:u32)
  n3 = local read "Time Resolution Per Bin(ns)"() -> (w4:u16)
  n4 = local read "Accumulation Delay(ns)"() -> (w2:u16)
  n5 = To Double Precision Float(number=w11) -> (double precision float=w10:dbl)
  n6 = To Double Precision Float(number=w6) -> (double precision float=w5:dbl)
  n7 = To Double Precision Float(number=w4) -> (double precision float=w7:dbl)
  n8 = To Double Precision Float(number=w2) -> (double precision float=w3:dbl)
  n9 = To Double Precision Float(number=1000000000) -> (double precision float=w8:dbl)
  n10 = Multiply(x=w5, y=w7) -> (x*y=w15:dbl)
  n11 = Add(x=w15, y=w3) -> (x+y=w14:dbl)
  n12 = Multiply(x=w10, y=w14) -> (x*y=w13:dbl)
  n13 = property on="Data Reads" class="DigNum (strict)"("Value"=0 ("Data Reads")) -> ()  [unwired: 2 in, 2 out]
  n14 = Divide(x=w13, y=w8) -> (x/y=w12:dbl)
  "Data Collection Time per Column" <- w12
  n15 = stacked-sequence {
    tunnel: w12 -> [_ _ _ _ w90 _]
    frame #0 {
      # "Closes Any Open Cards\nAnd Resets Indicators\nOn Front Panel"
      n16 = dll-call lib="AmcsUsb.dll" fn="_AMCSUSB_Close_All" label="Close_All"() -> ()  [unwired: 4 in, 2 out]
      "Open?" <- FALSE ("Open?")
      "Device ID" <- u32 0 ("Device ID")
      "Running?" <- FALSE ("Running?")
    }
    frame #1 {
      # "Responsible For Opening\nAnd Closing The Card"
      n17 = local read "Device ID"() -> (w20:u32)
      n18 = Equal To 0?(x=w20) -> (x = 0?=w19:bool)
      n19 = case shown="True" w19 {
        frame True {
          # "Opens Device"
          n20 = stacked-sequence {
            frame #0 {
              n21 = Decimal String To Number(string="0" ("Device Number")) -> (number=w21:i32)  [unwired: 2 in, 1 out]
              n22 = dll-call lib="AmcsUsb.dll" fn="AMCSUSB_Open"("devnum"=w21) -> ("return type"=w22:u32)  [unwired: 4 in, 2 out]
              n23 = local write "Device ID"(w22) -> ()
            }
            frame #1 {
              n24 = local read "Device ID"() -> (w24:u32)
              n25 = dll-call lib="AmcsUsb.dll" fn="_AMCSUSB_Reset" label="Reset"("handle"=w24) -> ()  [unwired: 5 in, 2 out]
            }
            frame #2 {
              n26 = local read "Device ID"() -> (w25:u32)
              n27 = Equal To 0?(x=w25) -> (x = 0?=w26:bool)
              n28 = case shown="False" w26 {
                frame False {
                  n29 = local write "Open?"(TRUE ("Open?")) -> ()
                }
                frame True {
                  n30 = local write "Open?"(FALSE ("Open?")) -> ()
                }
              }
            }
          }
        }
        frame False {
          # "Closes Device"
          n31 = dll-call lib="AmcsUsb.dll" fn="_AMCSUSB_Close_All" label="Close_All"() -> ()  [unwired: 4 in, 2 out]
          n32 = local write "Device ID"(u32 0 ("Device ID")) -> ()
        }
      }
    }
    frame #2 {
      # "Responsible For Setting\nThe Registers Of The\nCard And Running It"
      n33 = local read "Running?"() -> (w32:bool)
      n34 = local read "Open?"() -> (w33:bool)
      n35 = Not(x=w32) -> (.not. x?=w31:bool)
      n36 = And(x=w33, y=w31) -> (x .and. y?=w30:bool)
      n37 = case shown="True" w30 {
        frame False {
        }
        frame True {
          n38 = stacked-sequence {
            frame #0 {
              # "Sets The Registers Of The Card"
              # "Number Of Channels Used"
              n39 = expression code="x/10"("Time Resolution Per Bin(ns)") -> (w37:u16)
              n40 = expression code="x/80"("Pulse A Delay(ns)") -> (w39:u32)
              n41 = expression code="x/80"("Pulse B Delay(ns)") -> (w60:u32)
              n42 = expression code="x/10"("Accumulation Delay(ns)") -> (w41:u16)
              n43 = expression code="x*4"("Sync Pulse Polarity") -> (w46:enum32{"Low", "High"})
              n44 = expression code="x*2"("Pulse A Polarity") -> (w45:enum16{"Low", "High"})
              n45 = expression code="(x-1)*256"(u32 4 ("Number of Channels Used")) -> (w54:u32)
              n46 = To Unsigned Long Integer(number=w46) -> (unsigned 32bit integer=w47:u32)
              n47 = To Unsigned Long Integer(number=w45) -> (unsigned 32bit integer=w44:u32)
              n48 = To Unsigned Long Integer(number="Pulse B Polarity") -> (unsigned 32bit integer=w42:u32)
              n49 = To Unsigned Long Integer(number=w37) -> (unsigned 32bit integer=w36:u32)
              n50 = To Unsigned Long Integer(number=w39) -> (unsigned 32bit integer=w38:u32)
              n51 = To Unsigned Long Integer(number=w41) -> (unsigned 32bit integer=w40:u32)
              n52 = Compound Arithmetic op=ADD(w47, w44, w42, w54) -> (w59:u32)
              n53 = Build Array(w59, "Number of Bins", "Number of Accumulates", w36, w38, w60, w40) -> (w35:u32[])
              n54 = local read "Device ID"() -> (w52:u32)
              n55 = To Unsigned Word Integer(number=w35) -> (unsigned 16bit integer=w34:u16[])
              n56 = local write "ns scale"("Time Resolution Per Bin(ns)") -> ()
              n57 = local write "y offset"("Accumulation Delay(ns)") -> ()
              n58 = local write "bins"("Number of Bins") -> ()
              n59 = dll-call lib="AmcsUsb.dll" fn="_AMCSUSB_Write_Registers" label="Write_Registers"("handle"=w52, "registers"=w34) -> ()  [unwired: 6 in, 2 out]
            }
            frame #1 {
              # "Resets Buffers Of Card"
              n60 = local read "Device ID"() -> (w61:u32)
              n61 = dll-call lib="AmcsUsb.dll" fn="_AMCSUSB_Reset_FIFOs" label="Reset_FIFOs"("handle"=w61) -> ()  [unwired: 5 in, 2 out]
            }
            frame #2 {
              # "Starts Card Collecting Data"
              n62 = local read "Device ID"() -> (w62:u32)
              n63 = dll-call lib="AmcsUsb.dll" fn="_AMCSUSB_Go" label="Go"("handle"=w62) -> ()  [unwired: 5 in, 2 out]
            }
            frame #3 {
              n64 = local write "Running?"(TRUE) -> ()
            }
          }
        }
      }
    }
    frame #3 {
      # "Sets The Y-Scale Of The\nChart To Be In Selected\nUnits"
      n65 = stacked-sequence {
        frame #0 {
          # "Calculates A Recommended Minimum\nSync Pulse Period(sometimes incorrect\nwork in extreme situations)"
          n66 = local read "Time Resolution Per Bin(ns)"() -> (w71:u16)
          n67 = local read "Accumulation Delay(ns)"() -> (w73:u16)
          n68 = local read "Number of Bins"() -> (w72:u32)
          n69 = To Double Precision Float(number=w72) -> (double precision float=w74:dbl)
          n70 = To Double Precision Float(number=w71) -> (double precision float=w75:dbl)
          n71 = To Double Precision Float(number=w73) -> (double precision float=w76:dbl)
          n72 = Multiply(x=w74, y=w75) -> (x*y=w70:dbl)
          n73 = Add(x=w70, y=w76) -> (x+y=w68:dbl)
          n74 = Divide(x=w68, y=1000.0) -> (x/y=w67:dbl)
          n75 = Add(x=w67, y=1.0) -> (x+y=→"Minimum Sync Pulse Period(µs)":dbl)
        }
        frame #1 {
          n76 = local read "Minimum Sync Pulse Period(µs)"() -> (w78:dbl)
          n77 = Divide(x=w78, y=1000000.0) -> (x/y=w77:dbl)
          n78 = Reciprocal(x=w77) -> (1/x=→"Max. Rep. Rate (Hz)":dbl)
        }
      }
      n79 = case shown="0, Default" "y units" {
        frame 0, Default {
          (unwired) u8 0 ("Y Scale.Format & Precision:Precision")
          (unwired) u16 1 ("Y Scale.Offset and Multiplier:Multiplier")
          (unwired) "Bin #" ("Y Scale.Name Label.Text")
          (unwired) u16 0 ("Y Scale.Offset and Multiplier:Offset")
        }
        frame 1 {
          (unwired) u8 1 ("Y Scale.Format & Precision:Precision")
          (unwired) "Sample Time(µs)" ("Y Scale.Name Label.Text")
          n80 = local read "y offset"() -> (w84:u16)
          n81 = local read "ns scale"() -> (w83:u16)
          n82 = To Double Precision Float(number=w84) -> (double precision float=w82:dbl)
          n83 = To Double Precision Float(number=w83) -> (double precision float=w81:dbl)
          n84 = expression code="x/1000"(w82) -> ()  [unwired: 1 out]
          n85 = expression code="x/1000"(w81) -> ()  [unwired: 1 out]
        }
        frame 2 {
          (unwired) u8 0 ("Y Scale.Format & Precision:Precision")
          w85 = ext 0.299792458 ("y")
          (unwired) "Range(m)" ("Y Scale.Name Label.Text")
          n86 = local read "y offset"() -> (w88:u16)
          n87 = local read "ns scale"() -> (w89:u16)
          n88 = Multiply(x=w88, y=w85) -> (x*y=w87:ext)
          n89 = Multiply(x=w89, y=w85) -> (x*y=w86:ext)
          n90 = expression code="x/2"(w87) -> ()  [unwired: 1 out]
          n91 = expression code="x/2"(w86) -> ()  [unwired: 1 out]
        }
      }
    }
    frame #4 {
      n92 = while {
        tunnel: w90 -> [w93]
        i -> [w91]
        stop <- "stop" stop-if-true
        n93 = stacked-sequence {
          tunnel: w93 -> [w98 _]
          tunnel: [_ w99] -> _
          frame #0 {
            # "Delay loop?"
            n94 = To Double Precision Float(number=990) -> (double precision float=w96:dbl)
            n95 = Multiply(x=w98, y=w96) -> (x*y=w95:dbl)
            n96 = To Unsigned Long Integer(number=w95) -> (unsigned 32bit integer=w94:u32)
            n97 = Wait (ms)(milliseconds to wait=w94) -> ()  [unwired: 1 out]
          }
          frame #1 {
            n98 = local read "Running?"() -> (w100:bool)
            n99 = case shown="True" w100 {
              tunnel: [1 ("return type") w108] -> w99
              frame False {
              }
              frame True {
                w120 = 94 ("length")
                # "Collects Data From Card,\nSends It To The Chart"
                n100 = local read "bins"() -> (w125:u32)
                n101 = local read "Device ID"() -> (w133:u32)
                n102 = To Long Integer(number=w125) -> (32bit integer=w124:i32)
                n103 = local read "Number of Bins"() -> (w122:u32)
                n104 = dll-call lib="AmcsUsb.dll" fn="_AMCSUSB_DataStreamSize" label="DataStreamSize"("handle"=w133) -> ("return type"=w132:u16)  [unwired: 4 in, 2 out]
                n105 = expression code="x/2"(w132) -> (w131:u16)
                n106 = Subtract(x=w122, y=w120) -> (x-y=w121:u32)
                n107 = To Long Integer(number=w131) -> (32bit integer=w130:i32)
                n108 = Initialize Array(u32 0 ("element"), w130) -> (w134:u32[])
                n109 = dll-call lib="AmcsUsb.dll" fn="_AMCSUSB_ReadDataStream2" label="ReadDataStream2"("handle"=w133, "buffer"=w134, "BytesReturned"=u32 0) -> ("return type"=w108:i32, "buffer"=w126:u16[])  [unwired: 5 in, 2 out]
                "return type" <- w108
                n110 = stacked-sequence {
                  tunnel: w126 -> [w159 w176 w192 w208]
                  tunnel: w124 -> [w158 w164 w184 w200]
                  tunnel: [w147 _ _ _] -> w123
                  tunnel: [w146 _ _ _] -> w117
                  tunnel: w121 -> [w155 w172 w188 w204]
                  tunnel: w120 -> [w154 w173 w189 w205]
                  tunnel: [w152 _ _ _] -> w110
                  tunnel: "TC Start" -> [w151 w161 w177 w193]
                  tunnel: "TC Length" -> [w150 w162 w178 w194]
                  tunnel: [_ w170 _ _] -> w116
                  tunnel: [_ w167 _ _] -> w104
                  tunnel: [_ w166 _ _] -> w115
                  tunnel: [_ _ w181 _] -> w114
                  tunnel: [_ _ w180 _] -> w103
                  tunnel: [_ _ w179 _] -> w113
                  tunnel: [_ _ _ w197] -> w112
                  tunnel: [_ _ _ w196] -> w107
                  tunnel: [_ _ _ w195] -> w111
                  frame #0 {
                    n111 = Array Subset(array=w159, index=0 ("dimension size"), length=w158) -> (w156:u16[])
                    n112 = To Double Precision Float(number=w156) -> (double precision float=w149:dbl[])
                    n113 = Array Subset(array=w149, index=w155, length=w154) -> (w157:dbl[])
                    n114 = call-poly <vilib>:"Mean.vi"("X"=w157) -> ("mean"=w148:dbl)  [unwired: 1 out]
                    n115 = Array Subset(array=w149, index=w151, length=w150) -> (w153:dbl[])
                    n116 = Add Array Elements(numeric array=w153) -> (sum=w152:dbl)
                    n117 = To Double Precision Float(number=w149) -> (double precision float=w147:dbl[])
                    n118 = Subtract(x=w147, y=w148) -> (x-y=w146:dbl[])
                  }
                  frame #1 {
                    n119 = Multiply(x=w164, y=1 ("Far Input Ch")) -> (x*y=w163:i32)
                    n120 = Array Subset(array=w176, index=w163, length=w164) -> (w175:u16[])
                    n121 = To Double Precision Float(number=w175) -> (double precision float=w166:dbl[])
                    n122 = Array Subset(array=w166, index=w172, length=w173) -> (w174:dbl[])
                    n123 = call-poly <vilib>:"Mean.vi"("X"=w174) -> ("mean"=w168:dbl)  [unwired: 1 out]
                    n124 = To Double Precision Float(number=w166) -> (double precision float=w169:dbl[])
                    n125 = Array Subset(array=w166, index=w161, length=w162) -> (w171:dbl[])
                    n126 = Subtract(x=w169, y=w168) -> (x-y=w167:dbl[])
                    n127 = Add Array Elements(numeric array=w171) -> (sum=w170:dbl)
                  }
                  frame #2 {
                    n128 = Multiply(x=w184, y=2 ("Far Input Ch")) -> (x*y=w183:i32)
                    n129 = Array Subset(array=w192, index=w183, length=w184) -> (w191:u16[])
                    n130 = To Double Precision Float(number=w191) -> (double precision float=w179:dbl[])
                    n131 = Array Subset(array=w179, index=w188, length=w189) -> (w190:dbl[])
                    n132 = call-poly <vilib>:"Mean.vi"("X"=w190) -> ("mean"=w185:dbl)  [unwired: 1 out]
                    n133 = To Double Precision Float(number=w179) -> (double precision float=w186:dbl[])
                    n134 = Array Subset(array=w179, index=w177, length=w178) -> (w187:dbl[])
                    n135 = Subtract(x=w186, y=w185) -> (x-y=w180:dbl[])
                    n136 = Add Array Elements(numeric array=w187) -> (sum=w181:dbl)
                  }
                  frame #3 {
                    n137 = Multiply(x=w200, y=3 ("Far Input Ch")) -> (x*y=w199:i32)
                    n138 = Array Subset(array=w208, index=w199, length=w200) -> (w207:u16[])
                    n139 = To Double Precision Float(number=w207) -> (double precision float=w195:dbl[])
                    n140 = Array Subset(array=w195, index=w204, length=w205) -> (w206:dbl[])
                    n141 = call-poly <vilib>:"Mean.vi"("X"=w206) -> ("mean"=w201:dbl)  [unwired: 1 out]
                    n142 = To Double Precision Float(number=w195) -> (double precision float=w202:dbl[])
                    n143 = Array Subset(array=w195, index=w193, length=w194) -> (w203:dbl[])
                    n144 = Subtract(x=w202, y=w201) -> (x-y=w196:dbl[])
                    n145 = Add Array Elements(numeric array=w203) -> (sum=w197:dbl)
                  }
                }
                n146 = Equal To 0?(x=w108) -> (x = 0?=w109:bool)
                n147 = Multiply(x=w103, y="Near Ch Offline mult") -> (x*y=w102:dbl[])
                n148 = Multiply(x=w107, y="Near Ch Offline mult") -> (x*y=w106:dbl[])
                n149 = Build Array(w117, w104, w102, w106) -> (w129:dbl[][])
                n150 = Bundle(w110, w116, w114, w112) -> (w127:cluster{dbl, dbl, dbl, dbl})  [unwired: 1 in]
                n151 = Build Array(w123, w115, w113, w111) -> (w128:dbl[][])
                n152 = case shown="True" w109 {
                  tunnel: w129 -> [_ w145]
                  tunnel: w128 -> [_ w144]
                  tunnel: w127 -> [_ w143]
                  tunnel: w123 -> [_ w140]
                  tunnel: w115 -> [_ w139]
                  tunnel: w113 -> [_ w138]
                  tunnel: w111 -> [_ w137]
                  frame False {
                  }
                  frame True {
                    n153 = local read "Data Reads"() -> (w141:i32)
                    n154 = global write "Scalar_Data.vi" "Scalar Data"(w140) -> ()
                    n155 = global write "Scalar_Data.vi" "Scalar Data  2"(w139) -> ()
                    n156 = global write "Scalar_Data.vi" "Scalar Data  3"(w138) -> ()
                    n157 = global write "Scalar_Data.vi" "Scalar Data  4"(w137) -> ()
                    n158 = Increment(x=w141) -> (x+1=w142:i32)
                    n159 = local write "Data Reads"(w142) -> ()
                    "Corrected Return" <- w145
                    "Raw Uncorrected Return" <- w144
                    "Total Counts" <- w143
                  }
                }
              }
            }
          }
        }
        "Loop Count" <- w91
      }
    }
    frame #5 {
      # "Closes Any Open Cards\nAnd Resets Indicators\nOn Front Panel"
      n160 = dll-call lib="AmcsUsb.dll" fn="_AMCSUSB_Close_All" label="Close_All"() -> ()  [unwired: 4 in, 2 out]
      n161 = local write "Device ID"(u32 0 ("Device ID")) -> ()
      n162 = local write "Open?"(TRUE ("Open?")) -> ()
      n163 = local write "Running?"(FALSE ("Running?")) -> ()
    }
  }
